vi "FormatCommand.vi"(7 "CMD (MON)":u8(ring) items=["MON", "SET", "INFO"], 8 "VAL":string, 9 "PAR":string(combo)="BDNAME", 10 "CH":i8=-1 min=-1 max=4, 11 "BD (0)":i8 max=31) -> (3 "cmd":string)   [LabVIEW 2020, in "CAEN PSM.lvlib"]
uses:
  CAEN PSM.lvlib
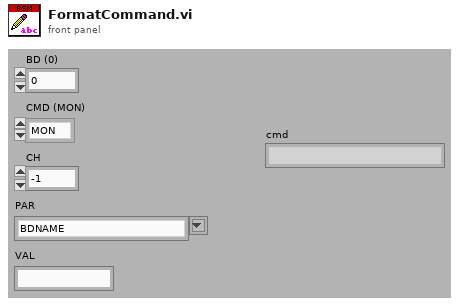
[diagram p1: front panel]
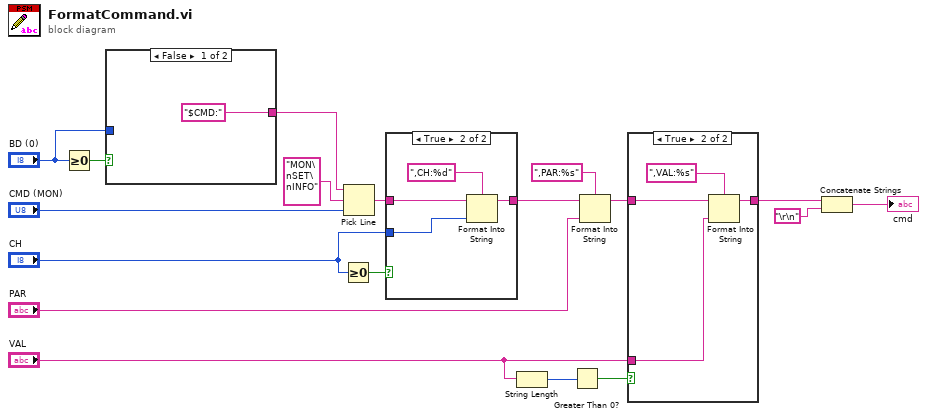
[diagram p0: block diagram]
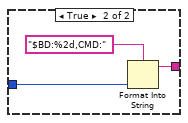
[diagram p2: hidden frame]
diagram:
  n1 = Greater Or Equal To 0?(x="BD (0)") -> (x >= 0?=w3:bool)
  n2 = case shown="False" w3 {
    tunnel: ["$CMD:" ("format string") w21] -> w2
    tunnel: "BD (0)" -> [_ w20]
    frame False {
    }
    frame True {
      n3 = Format Into String(format string="$BD:%2d,CMD:", w20) -> (resulting string=w21:string)  [unwired: 2 in, 1 out]
    }
  }
  n4 = Greater Or Equal To 0?(x="CH") -> (x >= 0?=w16:bool)
  n5 = Pick Line(string ("")=w2, multi-line string="MON\nSET\nINFO", line index="CMD (MON)") -> (output string=w14:string)
  n6 = case shown="True" w16 {
    tunnel: "CH" -> [_ w26]
    tunnel: w14 -> [w23 w25]
    tunnel: [w23 w24] -> w9
    frame False {
    }
    frame True {
      n7 = Format Into String(format string=",CH:%d", initial string=w25, w26) -> (resulting string=w24:string)  [unwired: 1 in, 1 out]
    }
  }
  n8 = String Length(string="VAL") -> (length=w13:i32)
  n9 = Greater Than 0?(x=w13) -> (x > 0?=w12:bool)
  n10 = Format Into String(format string=",PAR:%s", initial string=w9, "PAR") -> (resulting string=w7:string)  [unwired: 1 in, 1 out]
  n11 = case shown="True" w12 {
    tunnel: "VAL" -> [_ w31]
    tunnel: [w28 w30] -> w5
    tunnel: w7 -> [w28 w29]
    frame False {
    }
    frame True {
      n12 = Format Into String(format string=",VAL:%s", initial string=w29, w31) -> (resulting string=w30:string)  [unwired: 1 in, 1 out]
    }
  }
  n13 = Concatenate Strings(w5, "\r\n") -> (→"cmd":string)
